vi "Initialize.vi"(8 "error in":errorcluster, 11 "RDMA Transfer Rx User Interface in":refnum<class "RDMA Transfer Rx User Interface.lvclass">) -> (0 "error out":errorcluster, 3 "RDMA Transfer Rx User Interface out":refnum<class "RDMA Transfer Rx User Interface.lvclass">)   [LabVIEW 2020, in "RDMA.lvlib" / "RDMA Transfer Rx User Interface.lvclass"]
uses:
  RDMA Transfer Rx User Interface.lvclass
  Configuration/Rx Transfer/RDMA Transfer Rx Configuration.lvclass
  DSF Core.lvlibp/Classes/User Interface/User Interface.lvclass
  C:/srd-adg-hil/src/lruts/lruts_rdma/nivs-plugins-dirty/Components/DSF Core.lvlibp/Classes/Configuration/Configuration.lvclass
  C:/srd-adg-hil/src/lruts/lruts_rdma/nivs-plugins-dirty/Components/DSF Core.lvlibp/Classes/User Interface/User Interface.lvclass
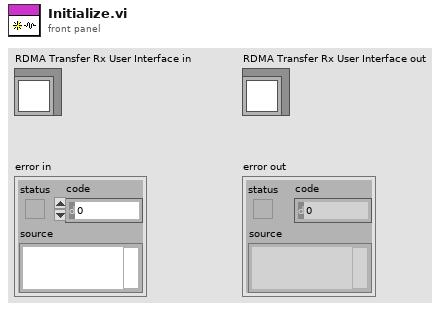
[diagram p1: front panel]
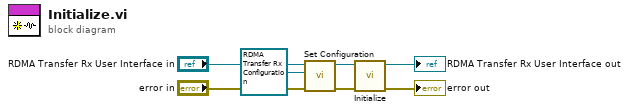
[diagram p0: block diagram]
diagram:
  n1 = call "Set Configuration.vi"("error in (no error)"="error in", "configuration"=refnum<class "RDMA Transfer Rx Configuration.lvclass"> refnum ("DSF Core.lvlib:UDP Transfer Rx Configuration.lvclass"), "User Interface in"="RDMA Transfer Rx User Interface in") -> ("error out"=w5:errorcluster, "User Interface out"=w4:refnum<class "RDMA Transfer Rx User Interface.lvclass">)  [unwired: 7 in]
  n2 = call-parent "Initialize.vi"("error in (no error)"=w5, "User Interface in"=w4) -> ("error out"=→"error out":errorcluster, "User Interface out"=→"RDMA Transfer Rx User Interface out":refnum<class "RDMA Transfer Rx User Interface.lvclass">)  [unwired: 8 in]
